vi "Remove Outliers.vi"   [LabVIEW 2014, in "NI_AALPro.lvlib"]
doc: "Removes data points that fall outside a given range or within a given index array. You must manually select the polymorphic instance you want to use."
uses:
  NI_AALPro.lvlib
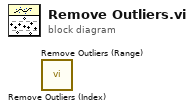
[diagram p0: block diagram]
diagram:
  n1 = call "Remove Outliers (Index).vi"() -> ()  [unwired: 12 in, 4 out]
  n2 = call "Remove Outliers (Range).vi"() -> ()  [unwired: 11 in, 5 out]
